vi "Handle48BitFIFOSetting.vi"(11 "FIFO value":u64) -> (3 "48 bit value":fxp<+,48,48>)   [LabVIEW 2018]
uses:
  <vilib>/rvi/FXPMathLib/FxpConvert/subVIs/nifxpmath_Convert_SimConfig.ctl
  <vilib>/fxp/LVFixedPointQuantizationPolicyTypeDef.ctl
  <vilib>/fxp/LVFixedPointOverflowPolicyTypeDef.ctl
  <vilib>/rvi/FXPMathLib/FxpConvert/simVIs/DllFxpConvertTemp_sub.vi
  <vilib>/rvi/FXPMathLib/FxpInterpret/XNode/nifxpmath_Interpret.xnode
  <vilib>/rvi/FXPMathLib/FxpConvert/XNode/nifxpmath_Convert.xnode
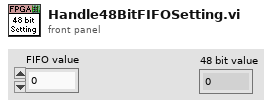
[diagram p1: front panel]
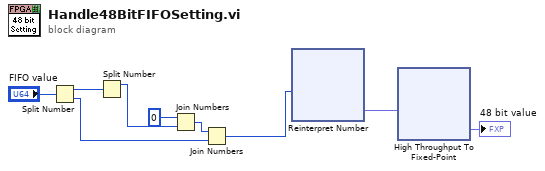
[diagram p0: block diagram]
diagram:
  n1 = Split Number(x="FIFO value") -> (hi(x)=w9:u32, lo(x)=w5:u32)
  n2 = Split Number(x=w9) -> (hi(x)=w8:u16)  [unwired: 1 out]
  n3 = Join Numbers(hi=u16 0, lo=w8) -> ((hi.lo)=w6:u32)
  n4 = Join Numbers(hi=w6, lo=w5) -> ((hi.lo)=w4:u64)
  n5 = xnode "Reinterpret Number"("x"=w4) -> ("y"=w3:fxp<+,64,64>)
  n6 = xnode "High Throughput To Fixed-Point"("x"=w3) -> ("y"=→"48 bit value":fxp<+,48,48>)
